vi "Display data.vi"(8 "Error in":errorcluster, 10 "Command":enum16{"Create", "Enqueue", "Dequeue", "Clear"}(ring), 11 "Data In":dbl[](array[numeric])) -> (0 "error out":errorcluster, 3 "Data out":dbl[](array[numeric]))   [LabVIEW 2016]
panel:
  # "Create: Khoi tao buffer\nEnqueue: Nap data vao buffer\nDequeue: Lay du lieu ra khoi buffer\nClear: Xoa toan bo buffer"
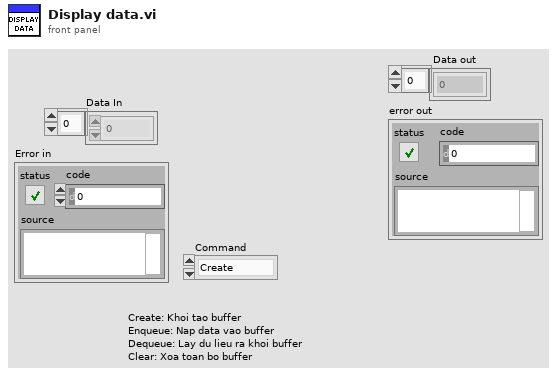
[diagram p1: front panel]
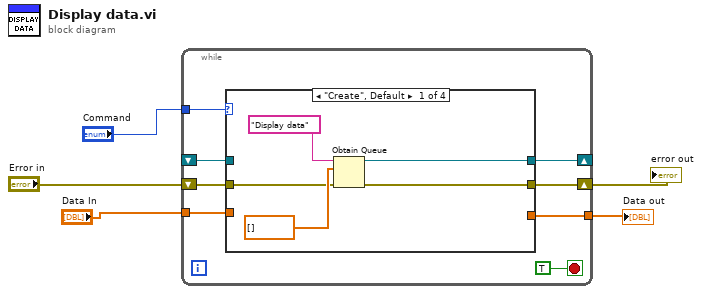
[diagram p0: block diagram]
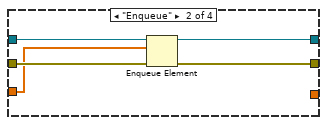
[diagram p2: hidden frame]
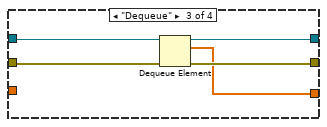
[diagram p3: hidden frame]
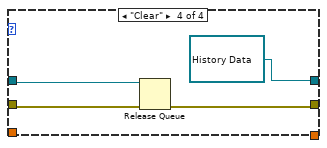
[diagram p4: hidden frame]
diagram:
  n1 = while {
    shift-right: [w12] -> _
    shift-left: _ -> [w11]
    shift-right: [w9] -> w1
    shift-left: "Error in" -> [w10]
    tunnel: "Data In" -> [w8]
    tunnel: [w7] -> w3
    tunnel: "Command" -> [w6]
    stop <- TRUE stop-if-true
    n2 = case shown="\"Create\", Default" w6 {
      tunnel: [w17 w20 w28 refnum<queue> refnum ("queue out")] -> w12
      tunnel: w11 -> [_ w23 w27 w32]
      tunnel: w10 -> [w15 w22 w26 w30]
      tunnel: [w14 w21 w25 w31] -> w9
      tunnel: w8 -> [_ w19 _ _]
      tunnel: [_ _ w24 _] -> w7
      frame "Create", Default {
        n3 = Obtain Queue(name (unnamed)="Display data", element data type=dbl[] [] ("History Data"), error in (no error)=w15) -> (queue out=w17:refnum<queue>, error out=w14:errorcluster)  [unwired: 2 in, 1 out]
      }
      frame "Enqueue" {
        n4 = Enqueue Element(queue=w23, element=w19, error in (no error)=w22) -> (queue out=w20:refnum<queue>, error out=w21:errorcluster)  [unwired: 1 in, 1 out]
      }
      frame "Dequeue" {
        n5 = Dequeue Element(queue=w27, error in (no error)=w26) -> (queue out=w28:refnum<queue>, element=w24:dbl[], error out=w25:errorcluster)  [unwired: 1 in, 1 out]
      }
      frame "Clear" {
        n6 = Release Queue(queue=w32, error in (no error)=w30) -> (error out=w31:errorcluster)  [unwired: 1 in, 2 out]
      }
    }
  }
  "Data out" <- w3
  "error out" <- w1
